vi "Dispose.vi"(8 "error in (no error)":errorcluster caption="错误输入（无错误）", 11 "Employee 输入":refnum<class "Employee.lvclass"> caption="DNL_LabVIEW Object in") -> (0 "error out":errorcluster caption="错误输出", 3 "Employee 输出":refnum<class "Employee.lvclass"> caption="DNL_LabVIEW Object out")   [LabVIEW 2012, in "Employee.lvclass"]
uses:
  Employee.lvclass
  Employee.lvclass/Employee.ctl
  Data Set/DataSet.lvclass
  Data Table/DataTable.lvclass
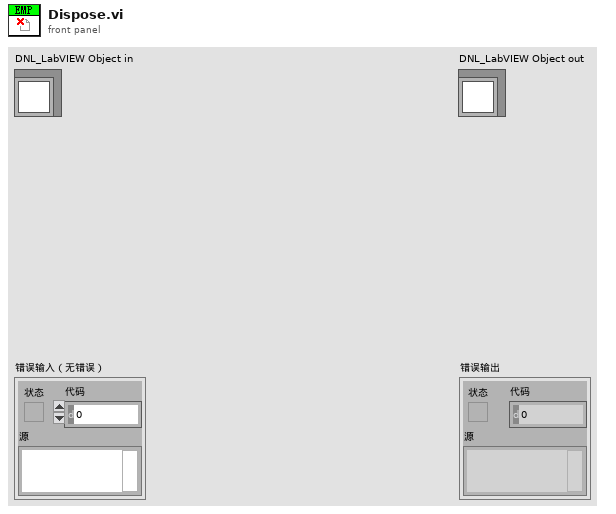
[diagram p1: front panel]
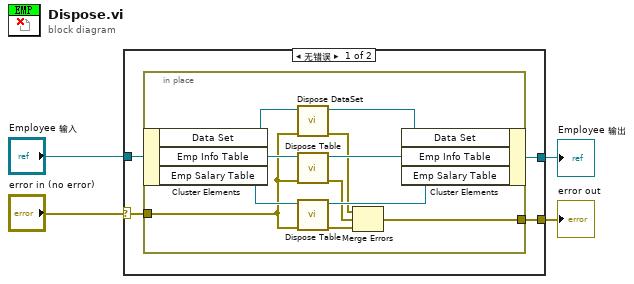
[diagram p0: block diagram]
diagram:
  n1 = case shown="无错误" "error in (no error)" {
    selector: "error in (no error)" -> [w7 w21]
    tunnel: [w6 w21] -> w3
    tunnel: [w5 w20] -> w1
    tunnel: "Employee 输入" -> [w8 w20]
    frame No Error {
      n2 = in-place {
        in-place-border: w7 -> [w13]
        in-place-border: [w9] -> w6
        n3 = in-place-cluster #1(w8) -> ("Data Set"=w15:refnum<class "DataSet.lvclass">, "Emp Info Table"=w19:refnum<class "DataTable.lvclass">, "Emp Salary Table"=w17:refnum<class "DataTable.lvclass">)
        n4 = call "Dispose DataSet.vi"("error in (no error)"=w13, "DataSet 输入"=w15) -> ("error out"=w12:errorcluster, "DataSet 输出"=w14:refnum<class "DataSet.lvclass">)  [unwired: 8 in]
        n5 = call "Dispose Table.vi"("error in (no error)"=w13, "DataTable 输入"=w19) -> ("error out"=w11:errorcluster, "DataTable 输出"=w18:refnum<class "DataTable.lvclass">)  [unwired: 8 in]
        n6 = call "Dispose Table.vi"("error in (no error)"=w13, "DataTable 输入"=w17) -> ("error out"=w10:errorcluster, "DataTable 输出"=w16:refnum<class "DataTable.lvclass">)  [unwired: 8 in]
        n7 = Merge Errors(w12, w11, w10) -> (w9:errorcluster)
        n8 = in-place-cluster #1("Data Set"=w14, "Emp Info Table"=w18, "Emp Salary Table"=w16) -> (w5:refnum<class "Employee.lvclass">)
      }
    }
    frame Error {
    }
  }
  "error out" <- w3
  "Employee 输出" <- w1
